vi "Add DPID.vi"(8 "error in (no error)":errorcluster, 11 "Node Ptr":u64 format="%.0x") -> (0 "error out":errorcluster)   [LabVIEW 2024, in "Diagnostics Addon System Explorer.lvlib"]
uses:
  Diagnostics Addon System Explorer.lvlib
  Addon Shared/Types/DPID.ctl
  Addon Shared/Types/DPID.Rate.ctl
  Types/FG.Action.ctl
  Addon Shared/Types/Type.ctl
  SubVIs/ID.FG.vi
  Addon Shared/SubVIs/Constants.vi
  <vilib>/NI VeriStand/Custom Device Tools/Custom Device Utility Library/NI VeriStand - Search for All Items by GUID.vi
  <vilib>/NI/NI VeriStand Advanced SysDef API/SysDef API/SysDef.Property.Set.vi
  <vilib>/NI/NI VeriStand Advanced SysDef API/_SubVIs/SysDef.Property.Set.U32.vi
  <vilib>/NI VeriStand/Custom Device API/NI VeriStand - Get Item Property.vi
  <vilib>/NI VeriStand/Custom Device API/Get Item Property (U32).vi
  <vilib>/NI/NI VeriStand Advanced SysDef API/_SubVIs/SysDef.Property.Set.U32.Array.vi
  <vilib>/NI VeriStand/Custom Device API/Get Item Property (U32 Array).vi
  Addon Shared/Diagnostics Addon Shared.lvlib
  <vilib>/NI VeriStand/Custom Device Tools/Custom Device Utility Library/Custom Device Utility Library.lvlib
panel:
  in  "Tag":string
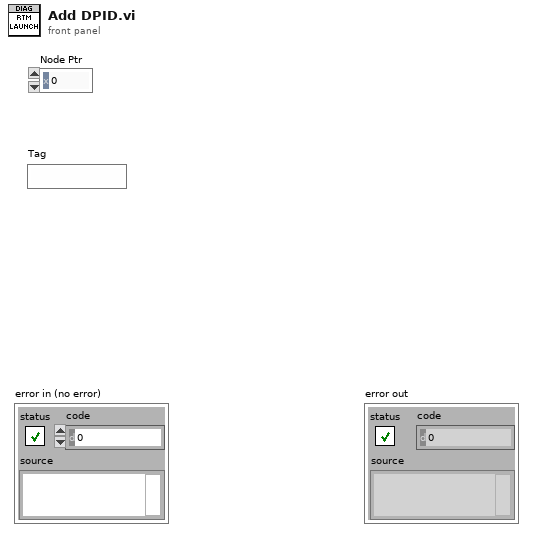
[diagram p1: front panel]
types:
  T1 = typedef "Diagnostics Addon Shared.lvlib/DPID.ctl" = cluster{"DPID ID":u8, "Speed":T2, "PIDs":u16[]}
  T2 = typedef "Diagnostics Addon Shared.lvlib/DPID.Rate.ctl" = enum16{"Slow", "Medium", "Fast"}
  T3 = typedef "Custom Device API.lvlib/Custom Device Item Ref.ctl" = u64
  T4 = typedef "Diagnostics Addon System Explorer.lvlib/FG.Action.ctl" = enum16{"Get", "Set"}
  T5 = typedef "Diagnostics Addon System Explorer.lvlib/Frame.Export.ctl" = cluster{"Name":string, "ID":u32, "Signals":T6[]}
  T6 = typedef "Diagnostics Addon Shared.lvlib/Signal.ctl" = cluster{"Start Bit":u32, "Length":u32, "Scaling Factor":dbl, "Scaling Offset":dbl, "Minimum":dbl, "Maximum":dbl, "Data Type":u32, "Byte Order":u32, "Default Value":dbl, "Name":string, "Units":string}
  T7 = typedef "Diagnostics Addon Shared.lvlib/Type.ctl" = enum16{"DID", "CDID", "PID", "CPID", "Read Memory", "Write Memory", "IO Control", "Routine Start", "Routine Request", "Routine Stop", "User Defined", "DTC Control", "Clear DTCs", "Read DTCs", "Start DTCs", "DTC Change Count", "Tester Present", "Unlock ECU", "Reset ECU", "Diag Session Control", "Communication Control", "DPID Control", "Poll Control", "Diag Comm Port Control"}
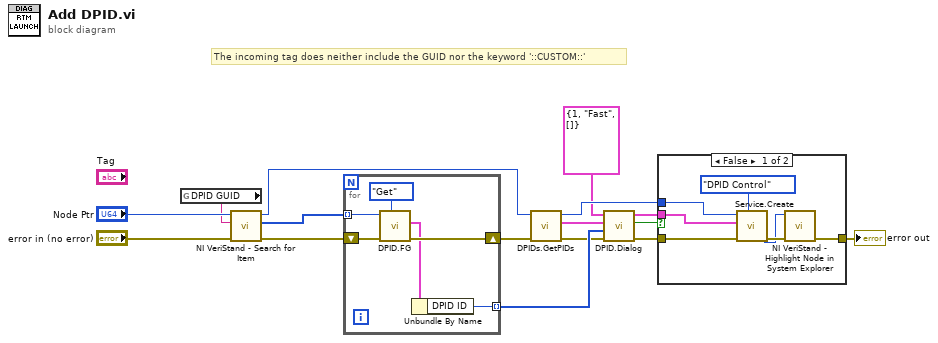
[diagram p0: block diagram]
diagram:
  # "The incoming tag does neither include the GUID nor the keyword '::CUSTOM::'"
  n1 = global read "Constants.vi" "DPID GUID"() -> (w2:string)
  n2 = call-poly <vilib>:"NI VeriStand - Search for Item.vi"("error in"="error in (no error)", "Item GUID"=w2, "Section Ref in"="Node Ptr") -> ("error out"=w12:errorcluster, "Item Refs"=w13:T3[], "Section Ref out"=w14:T3)  [unwired: 5 in, 1 out]
  n3 = for {
    tunnel: w13 -> [w22] mode=indexing
    shift-right: [w20] -> w11
    shift-left: w12 -> [w21]
    tunnel: [w18] -> w10 mode=indexing
    n4 = call "DPID.FG.vi"("Action"=FG.Action."Get", "error in (no error)"=w21, "Device Item Ref in"=w22) -> ("error out"=w20:errorcluster, "DPID"=w19:T1)  [unwired: 6 in, 1 out]
    n5 = Unbundle By Name(w19) -> ("DPID ID"=w18:u8)
  }
  n6 = call "DPIDs.GetPIDs.vi"("error in (no error)"=w11, "Item Ref in"=w14) -> ("error out"=w3:errorcluster, "PIDs"=w4:T5[], "Section Ref out"=w5:T3)  [unwired: 7 in]
  n7 = call "DPID.Dialog.vi"("error in (no error)"=w3, "Existing DPIDs"=w10, "Existing PIDs"=w4, "DPID"=T1 {"DPID ID"=1, "Speed"=enum."Fast", "PIDs"=[]}) -> ("error out"=w7:errorcluster, "Cancel PID?"=w9:bool, "DPID"=w8:T1)  [unwired: 5 in]
  n8 = case shown="False" w9 {
    tunnel: w8 -> [w28 _]
    tunnel: w7 -> [w24 w30]
    tunnel: [w29 w30] -> w6
    tunnel: w5 -> [w23 _]
    frame False {
      n9 = call "Service.Create.vi"("Type"=Type."DPID Control", "error in (no error)"=w24, "Variant"=w28, "Section Ptr"=w23) -> ("error out"=w27:errorcluster, "Parent Ref out"=w26:T3)  [unwired: 6 in]
      n10 = call <vilib>:"NI VeriStand - Highlight Node in System Explorer.vi"("error in (no error)"=w27, "Item Ref in"=w26) -> ("error out"=w29:errorcluster)  [unwired: 8 in, 1 out]
    }
    frame True {
    }
  }
  "error out" <- w6
